vi "Start Report.vi"(8 "error in (no error)":errorcluster {"code" format="Error %.0f"}, 11 "VIDoc Printer In":refnum<class "VIDoc Printer.lvclass">) -> (0 "error out":errorcluster {"code" format="Error %.0f"}, 3 "VIDoc Printer Out":refnum<class "VIDoc Printer.lvclass">)   [LabVIEW 2023, in "VIDoc Printer.lvlib" / "VIDoc Printer.lvclass"]
uses:
  VIDoc Printer.lvclass
  VIDoc Printer.lvclass/VIDoc Printer.ctl
  UI Interaction/Interface/UI Interaction.lvclass
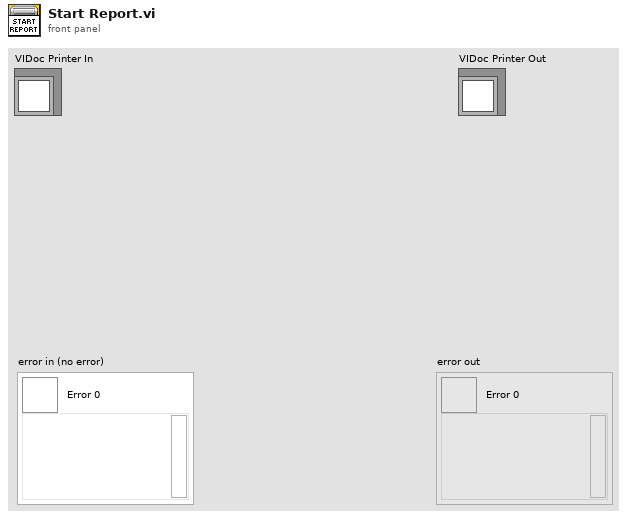
[diagram p1: front panel]
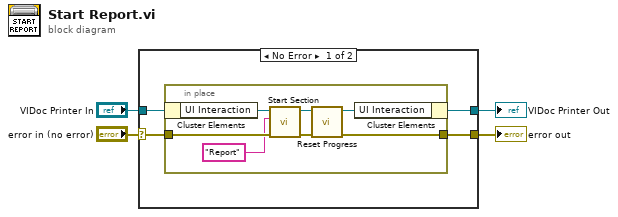
[diagram p0: block diagram]
diagram:
  n1 = case shown="No Error" "error in (no error)" {
    selector: "error in (no error)" -> [w6 w17]
    tunnel: [w5 w17] -> w3
    tunnel: [w8 w16] -> w1
    tunnel: "VIDoc Printer In" -> [w7 w16]
    frame No Error {
      n2 = in-place {
        in-place-border: w6 -> [w15]
        in-place-border: [w10] -> w5
        n3 = in-place-cluster #1(w7) -> ("UI Interaction"=w12:refnum<class "UI Interaction.lvclass">)
        n4 = call-dynamic "Start Section.vi"("error in (no error)"=w15, "Section"="Report", "UI Interaction in"=w12) -> ("error out"=w13:errorcluster, "UI Interaction out"=w14:refnum<class "UI Interaction.lvclass">)  [unwired: 7 in]
        n5 = call "Reset Progress.vi"("error in (no error)"=w13, "UI Interaction in"=w14) -> ("error out"=w10:errorcluster, "UI Interaction out"=w11:refnum<class "UI Interaction.lvclass">)  [unwired: 8 in]
        n6 = in-place-cluster #1("UI Interaction"=w11) -> (w8:refnum<class "VIDoc Printer.lvclass">)
      }
    }
    frame Error {
    }
  }
  "error out" <- w3
  "VIDoc Printer Out" <- w1
